vi "XY Graph Get Plot Data & Info.vi"(0 "Destination Graph":refnum<vi>, 5 "Original Graph":refnum<vi>, 7 "Original Plot Idx":i32=-1, 11 "Error In":errorcluster, 12 "Plot Style in":T2={"Plot Index"=0, "Plot.Bar Plot Style"=0, "Plot.DigitalLineStyle"=1, "Plot.TransitionLocation"=2, "Plot.Transition Type"=0, "Plot.Fill To"=-1, "Plot.Fill/Pt. Color"=16777222, "Plot.Label Format"=3, "Plot.Line Style"=0, "Plot.Line Width"=1, "Plot.Plot Color"=16777222, "Plot.Plot Interpolation"=2, "Plot.Plot Name"="", "Plot.Point Style"=0, "Plot.Visible?"=TRUE, "Plot.XScaleIdx"=0, "Plot.YScaleIdx"=0, "Plot.Anti-aliased"=TRUE}, 13 "Plot in":T1, 14 "Graph Origin Name":string) -> (3 "Refnum based call":bool, 4 "VI Title Suffix":string, 6 "X Array":dbl[](array[numeric]), 8 "Y Array":dbl[](array[numeric]), 10 "Plot Style out":T2, 15 "Error Out":errorcluster)   [LabVIEW 2019]
uses:
  XY Graph Plot Properties.ctl
  XY Plot Data.ctl
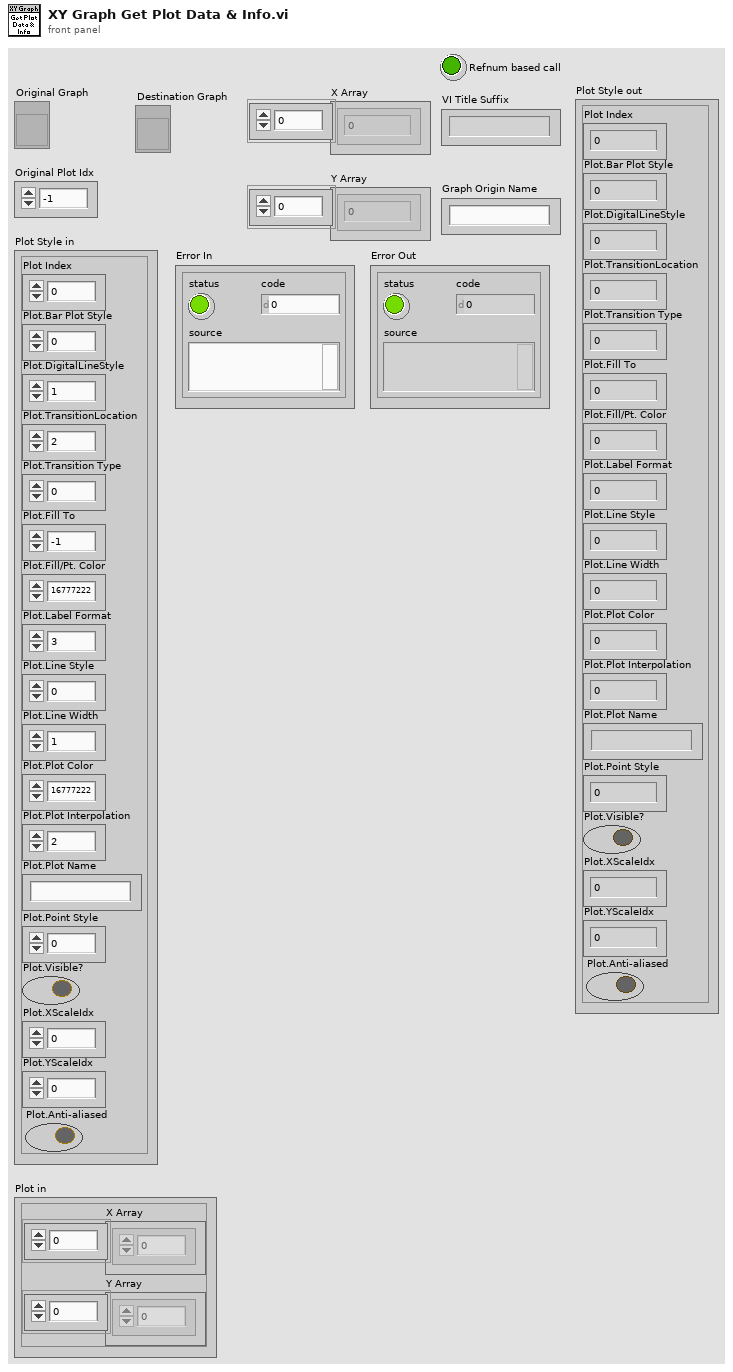
[diagram p1: front panel]
types:
  T1 = typedef "XY Plot Data.ctl" = cluster{"X Array":dbl[], "Y Array":dbl[]}
  T2 = typedef "XY Graph Plot Properties.ctl" = cluster{"Plot Index":i32, "Plot.Bar Plot Style":u8, "Plot.DigitalLineStyle":u8, "Plot.TransitionLocation":u8, "Plot.Transition Type":u8, "Plot.Fill To":i16, "Plot.Fill/Pt. Color":u32, "Plot.Label Format":u8, "Plot.Line Style":u8, "Plot.Line Width":u8, "Plot.Plot Color":u32, "Plot.Plot Interpolation":u8, "Plot.Plot Name":string, "Plot.Point Style":u8, "Plot.Visible?":bool, "Plot.XScaleIdx":u32, "Plot.YScaleIdx":u32, "Plot.Anti-aliased":bool}
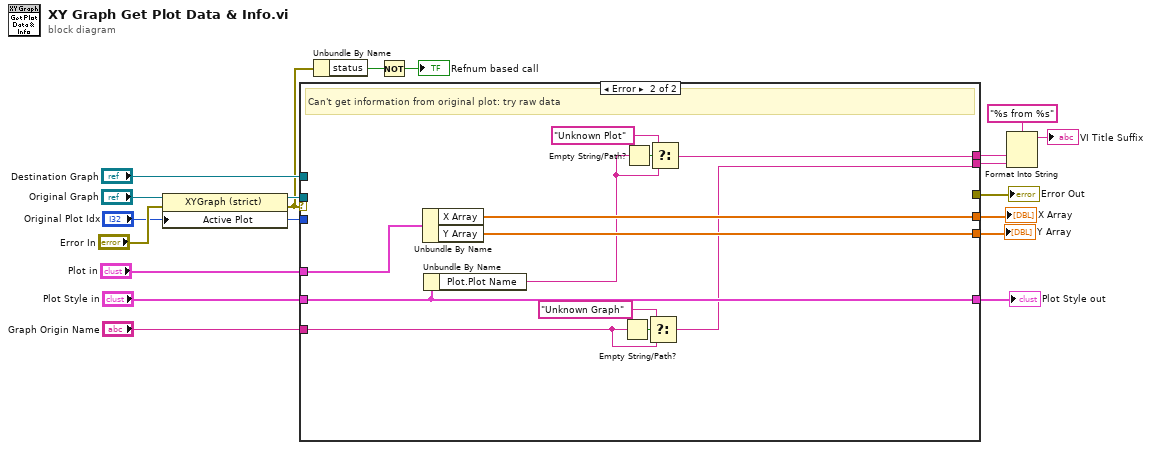
[diagram p0: block diagram]
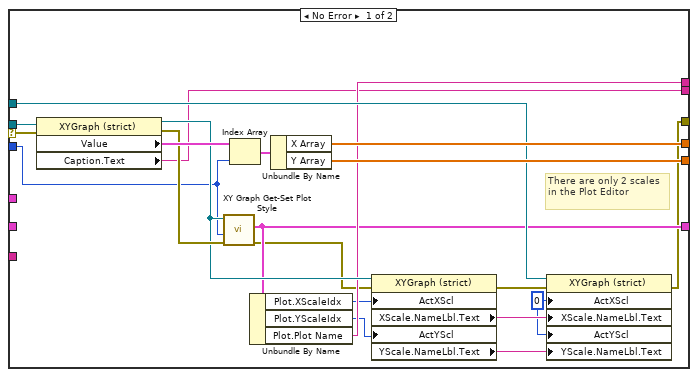
[diagram p2: hidden frame]
diagram:
  n1 = property class="XYGraph (strict)"(reference="Original Graph", error in="Error In", "Active Plot"="Original Plot Idx") -> (reference out=w12:refnum<vi>, error out=w3:errorcluster)
  n2 = case shown="Error" w3 {
    selector: w3 -> [w22 _]
    tunnel: "Plot in" -> [_ w52]
    tunnel: [w37 w51] -> w17
    tunnel: [w36 w50] -> w16
    tunnel: "Plot Style in" -> [_ w49]
    tunnel: [w23 w49] -> w14
    tunnel: w12 -> [w40 _]
    tunnel: "Original Plot Idx" -> [w25 _]
    tunnel: [w20 _] -> w10
    tunnel: "Destination Graph" -> [w32 _]
    tunnel: [w30 w47] -> w6
    tunnel: [w29 w44] -> w5
    tunnel: "Graph Origin Name" -> [_ w43]
    frame No Error {
      w24 = 0 ("Active X Scale")
      # "There are only 2 scales in the Plot Editor"
      n3 = property class="XYGraph (strict)"(reference=w40, error in=w22) -> (reference out=w34:refnum<vi>, error out=w35:errorcluster, "Value"=w39:cluster{"X Array":dbl[], "Y Array":dbl[]}[], "Caption.Text"=w29:string)
      n4 = call "XY Graph Get-Set Plot Style.vi"("Error In"=w35, "Plot Index"=w25, "XYGraph in"=w34) -> ("Error Out"=w21:errorcluster, "Plot Style out"=w23:T2)  [unwired: 5 in, 2 out]
      n5 = Index Array(array=w39, index=w25) -> (element=w38:cluster{"X Array":dbl[], "Y Array":dbl[]})
      n6 = Unbundle By Name(w23) -> ("Plot.XScaleIdx"=w27:u32, "Plot.YScaleIdx"=w26:u32, "Plot.Plot Name"=w30:string)
      n7 = Unbundle By Name(w38) -> ("X Array"=w37:dbl[], "Y Array"=w36:dbl[])
      n8 = property class="XYGraph (strict)"(reference=w34, error in=w21, "ActXScl"=w27, "ActYScl"=w26) -> (error out=w31:errorcluster, "XScale.NameLbl.Text"=w28:string, "YScale.NameLbl.Text"=w33:string)  [unwired: 1 out]
      n9 = property class="XYGraph (strict)"(reference=w32, error in=w31, "ActXScl"=w24, "XScale.NameLbl.Text"=w28, "ActYScl"=w24, "YScale.NameLbl.Text"=w33) -> (error out=w20:errorcluster)  [unwired: 1 out]
    }
    frame Error {
      # "Can't get information from original plot: try raw data"
      n10 = Unbundle By Name(w52) -> ("X Array"=w51:dbl[], "Y Array"=w50:dbl[])
      n11 = Unbundle By Name(w49) -> ("Plot.Plot Name"=w46:string)
      n12 = Empty String/Path?(string/path=w43) -> (empty?=w45:bool)
      n13 = Empty String/Path?(string/path=w46) -> (empty?=w48:bool)
      n14 = Select(t="Unknown Graph", s=w45, f=w43) -> (s? t:f=w44:string)
      n15 = Select(t="Unknown Plot", s=w48, f=w46) -> (s? t:f=w47:string)
    }
  }
  "Plot Style out" <- w14
  "Y Array" <- w16
  "X Array" <- w17
  "Error Out" <- w10
  n16 = Unbundle By Name(w3) -> ("status"=w2:bool)
  n17 = Not(x=w2) -> (.not. x?=→"Refnum based call":bool)
  n18 = Format Into String(format string="%s from %s", w6, w5) -> (resulting string=→"VI Title Suffix":string)  [unwired: 2 in, 1 out]
